vi "Check Tx Async Execution Unit Message Count.vi"(7 "Triggerable Frames Count":i32, 8 "error in":errorcluster, 9 "shared resources in":refnum<class "Shared Resources.lvclass">, 10 "Execution Unit":refnum<class "Execution Unit.lvclass">, 11 "Create Execution Unit in":refnum<class "Create Execution Unit.lvclass">) -> (0 "error out":errorcluster, 1 "shared resources out":refnum<class "Shared Resources.lvclass">, 3 "Create Execution Unit out":refnum<class "Create Execution Unit.lvclass">)   [LabVIEW 2020, in "Create Execution Unit.lvclass"]
uses:
  Create Execution Unit.lvclass
  Engine/Implementation/Shared Resources/Shared Resources.lvclass
  C:/Users/nitest/Desktop/Git 2020/niveristand-aim-milStd1553-custom-device/Source/Custom Device Support/Engine/Interfaces/Shared Resources/Shared Resources.lvclass
  Engine/Interfaces/Execution Unit/Execution Unit.lvclass
  Engine/Implementation/Tx Acyclic Execution Unit/Tx Acyclic Execution Unit.lvclass
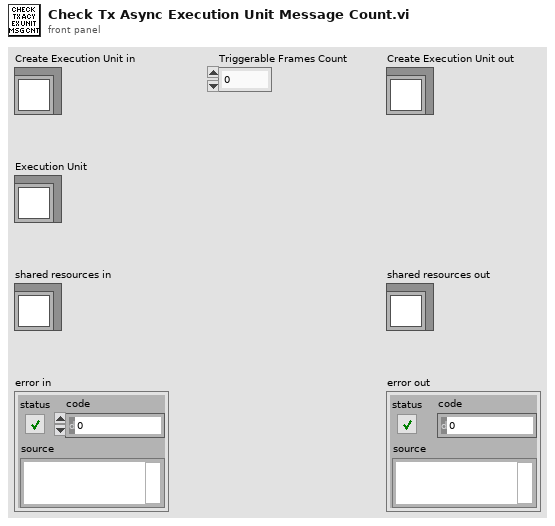
[diagram p1: front panel]
types:
  T1 = typedef "AIM MIL-STD-1553 Engine.lvlib/Implementation.lvlib/Tx Acyclic Execution Unit.lvclass/Triggerable Frame.ctl" = cluster{"Acyclic Transfer IDs":u16[], "Acyclic Messages":T2[]}
  T2 = typedef "AIM MIL-STD-1553 Engine.lvlib/Custom Device.lvlib/Compiled Message.ctl" = cluster{"Message Section Handle":T3, "First Parameter Index":i32, "Parameter Channel Handles":T3[], "Direction":T4, "Parameters":T5[], "Receiving RT Address":u8, "Receiving RT Sub-address":u8, "Transmitting RT Address":u8, "Transmitting RT Sub-address":u8, "Word Count":u8, "Buffer Type":enum16{"unknown", "BC Message Buffer", "RT Message Buffer"}, "Buffer ID":u16, "Terminal Type":enum16{"Bus Controller", "Remote Terminal"}, "Timestamp Enabled":bool, "Timestamp Channel Handle":T3}
  T3 = typedef "Custom Device API.lvlib/Custom Device Item Ref.ctl" = u64
  T4 = typedef "Direction.ctl" = enum16{"Rx", "Tx"}
  T5 = typedef "Parameter Definition.ctl" = cluster{"start index":i32, "size (bits)":i32, "encoding":enum16{"BNR", "BCD", "Discrete"}, "signed":bool, "multiplier":dbl, "offset":dbl}
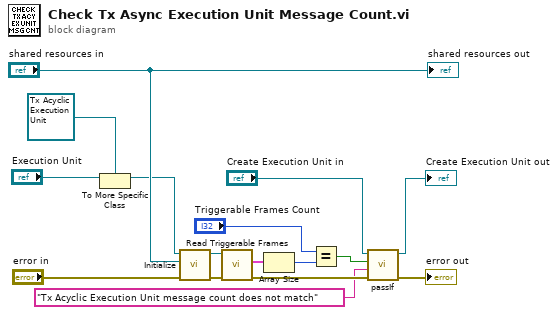
[diagram p0: block diagram]
diagram:
  n1 = To More Specific Class(target class=refnum<class "Tx Acyclic Execution Unit.lvclass"> refnum ("Address Based Execution Unit Implementation in"), reference="Execution Unit") -> (specific class reference=w3:refnum<class "Tx Acyclic Execution Unit.lvclass">)  [unwired: 1 in, 1 out]
  n2 = call-dynamic "Initialize.vi"("error in"="error in", "shared resources"="shared resources in", "tx acyclic execution unit"=w3) -> ("error out"=w5:errorcluster, "tx acyclic execution unit out"=w6:refnum<class "Tx Acyclic Execution Unit.lvclass">)  [unwired: 7 in]
  n3 = call-dynamic "Read Triggerable Frames.vi"("error in (no error)"=w5, "Tx Acyclic Execution Unit in"=w6) -> ("error out"=w13:errorcluster, "Triggerable Frames"=w8:T1[])  [unwired: 7 in, 1 out]
  n4 = Array Size(array=w8) -> (size(s)=w7:i32)
  n5 = Equal?(x="Triggerable Frames Count", y=w7) -> (x = y?=w15:bool)
  n6 = call-dynamic "passIf.vi"("error in (no error)"=w13, "message (\"\")"="Tx Acyclic Execution Unit message count does not match" ("message (\"\")"), "pass"=w15, "TestCase in"="Create Execution Unit in") -> ("error out"=→"error out":errorcluster, "TestCase out"=→"Create Execution Unit out":refnum<class "Create Execution Unit.lvclass">)  [unwired: 6 in]
  "shared resources out" <- "shared resources in"
